vi "create htm file.vi"(2 "last mod":timestamp, 3 "Source path":path, 4 "Destination path":path) -> ()   [LabVIEW 2010]
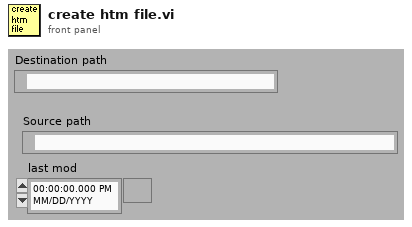
[diagram p1: front panel]
types:
  T1 = enum16{"open", "open or create", "create or replace", "create", "open (read only)"}
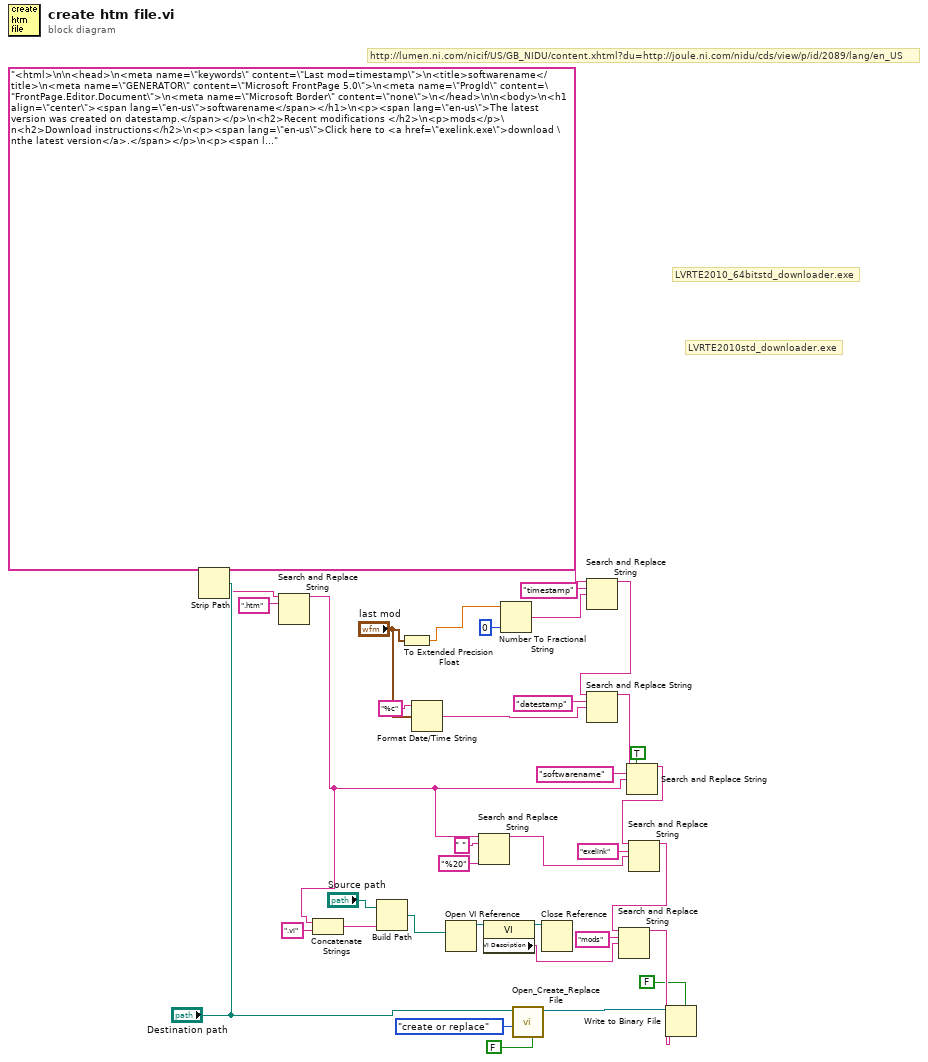
[diagram p0: block diagram]
diagram:
  # "LVRTE2010std_downloader.exe"
  # "LVRTE2010_64bitstd_downloader.exe"
  # "http://lumen.ni.com/nicif/US/GB_NIDU/content.xhtml?du=http://joule.ni.com/nidu/cds/view/p/id/2089/lang/en_US"
  n1 = Strip Path(path="Destination path") -> (name=w33:string)  [unwired: 1 out]
  n2 = Search and Replace String(input string=w33, search string=".htm") -> (result string=w6:string)  [unwired: 6 in, 3 out]
  n3 = Concatenate Strings(w6, ".vi" ("string")) -> (w4:string)
  n4 = Build Path(base path="Source path", name or relative path=w4) -> (appended path=w7:path)
  n5 = To Extended Precision Float(1:"last mod") -> (0:w14:ext)
  n6 = Format Date/Time String(time format string (%c)="%c", seconds (now)="last mod") -> (date/time string=w18:string)  [unwired: 1 in]
  n7 = Open VI Reference(vi path=w7) -> (vi reference=w12:refnum<vi>)  [unwired: 5 in, 1 out]
  n8 = Search and Replace String(input string=w6, search string=" ", replace string="%20" ("replace string (\"\")")) -> (result string=w24:string)  [unwired: 5 in, 3 out]
  n9 = property class="VI"(reference=w12) -> (reference out=w11:refnum<vi>, "VI Description"=w9:string)  [unwired: 1 in, 1 out]
  n10 = Number To Fractional String(number=w14, precision (6)=i16 0) -> (F-format string=w13:string)  [unwired: 2 in]
  n11 = call <vilib>:"Open_Create_Replace File.vi"("advisory dialog? (display:T)"=FALSE, "function (open:0)"=T1."create or replace", "file path"="Destination path") -> ("refnum"=w35:refnum<file>)  [unwired: 5 in, 3 out]
  n12 = Close Reference(reference=w11) -> ()  [unwired: 1 in, 1 out]
  n13 = Search and Replace String(input string="<html>\n\n<head>\n<meta name=\"keywords\" content=\"Last mod=timestamp\">\n<title>softwarename</title>\n<meta name=\"GENERATOR\" content=\"Microsoft FrontPage 5.0\">\n<meta name=\"ProgId\" content=\"FrontPage.Editor.Document\">\n<meta name=\"Microsoft Border\" content=\"none\">\n</head>\n\n<body>\n<h1 align=\"center\"><span lang=\"en-us\">softwarename</span></h1>\n<p><span lang=\"en-us\">The latest version was created on datestamp.</span></p>\n<h2>Recent modifications </h2>\n<p>mods</p>\n<h2>Download instructions</h2>\n<p><span lang=\"en-us\">Click here to <a href=\"exelink.exe\">download \nthe latest version</a>.</span></p>\n<p><span lang=\"en-us\">This software requires </span>LabVIEW Runtime\n<span lang=\"en-us\">available from the</span>\n<a href=\"LVRTE2010std_downloader.exe\">National Instruments \n site</a>.</p>\n<p><span lang=\"en-us\">If this application communicates with an instrument then \nit will require the VISA Runtime available from\n<a href=\"http://digital.ni.com/softlib.nsf/webcategories/85256410006C055586256BAC002C51FA?opendocument\">\nNational Instruments VISA download site</a>.</span></p>\n<p><span lang=\"en-us\"></li>\n</ul>\n</body>\n</html>", search string="timestamp", replace string=w13) -> (result string=w23:string)  [unwired: 5 in, 3 out]
  n14 = Search and Replace String(input string=w23, search string="datestamp", replace string=w18) -> (result string=w22:string)  [unwired: 5 in, 3 out]
  n15 = Search and Replace String(replace all?=TRUE ("replace all? (F)"), input string=w22, search string="softwarename", replace string=w6) -> (result string=w26:string)  [unwired: 4 in, 3 out]
  n16 = Search and Replace String(input string=w26, search string="exelink", replace string=w24) -> (result string=w2:string)  [unwired: 5 in, 3 out]
  n17 = Search and Replace String(input string=w2, search string="mods", replace string=w9) -> (result string=w3:string)  [unwired: 5 in, 3 out]
  n18 = Write to Binary File(file (use dialog)=w35, data=w3, 5:FALSE ("prepend array or string size? (T)")) -> ()  [unwired: 3 in, 3 out]
